vi "Convert array of NOK tests to text for display.vi"(11 "NOK tests from previous DUT":string[](array[string])) -> (3 "Text for display":string)   [LabVIEW 2023, in "In a row NOK.lvlib"]
uses:
  In a row NOK.lvlib
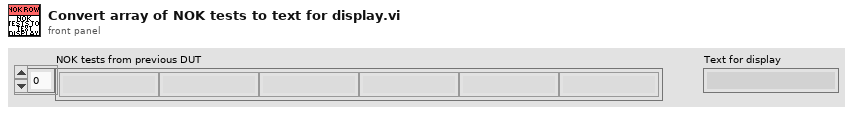
[diagram p1: front panel]
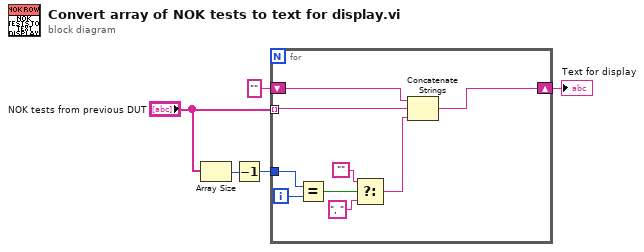
[diagram p0: block diagram]
diagram:
  n1 = Array Size(array="NOK tests from previous DUT") -> (size(s)=w2:i32)
  n2 = Decrement(x=w2) -> (x-1=w1:i32)
  n3 = for {
    tunnel: "NOK tests from previous DUT" -> [w13] mode=indexing
    shift-right: [w12] -> w5
    shift-left: "" -> [w14]
    tunnel: w1 -> [w11]
    i -> [w10]
    n4 = Equal?(x=w11, y=w10) -> (x = y?=w9:bool)
    n5 = Select(t="", s=w9, f=", ") -> (s? t:f=w6:string)
    n6 = Concatenate Strings(w14, w13, w6) -> (w12:string)
  }
  "Text for display" <- w5
